vi "Unblacklist Channel.vi"(8 "error in (no error)":errorcluster, 9 "Channel 2":string, 10 "Channel 1":string, 11 "SLSC Switch in":refnum<class "SLSC Switch.lvclass">) -> (0 "error out":errorcluster, 1 "found?":bool, 3 "SLSC Switch out":refnum<class "SLSC Switch.lvclass">)   [LabVIEW 2015, in "SLSC Switch.lvclass"]
uses:
  SLSC Switch.lvclass
  SLSC Switch.lvclass/SLSC Switch.ctl
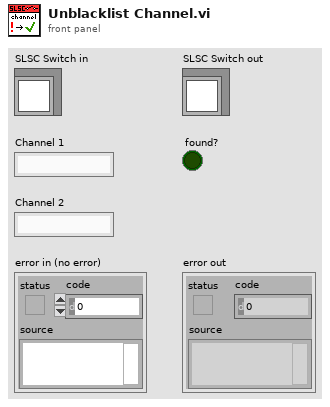
[diagram p1: front panel]
types:
  T1 = typedef "SLSC Switch.lvclass/Connection.ctl" = cluster{"channel 1":string, "channel 2":string}
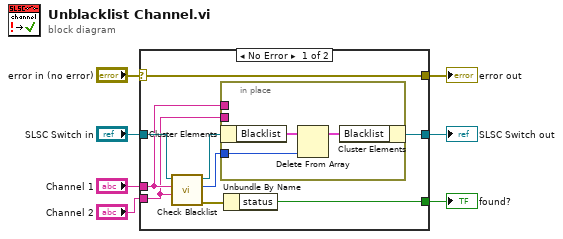
[diagram p0: block diagram]
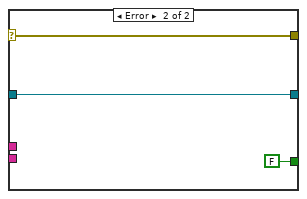
[diagram p2: hidden frame]
diagram:
  n1 = case shown="No Error" "error in (no error)" {
    selector: "error in (no error)" -> [w16 w22]
    tunnel: [w16 w22] -> w6
    tunnel: [w15 w21] -> w4
    tunnel: "SLSC Switch in" -> [w14 w21]
    tunnel: "Channel 1" -> [w12 _]
    tunnel: [w8 FALSE] -> w2
    tunnel: "Channel 2" -> [w11 _]
    frame No Error {
      n2 = call "Check Blacklist.vi"("Channel 2"=w11, "Channel 1"=w12, "SLSC Switch in"=w14) -> ("error out"=w9:errorcluster, "index"=w10:i32, "SLSC Switch out"=w13:refnum<class "SLSC Switch.lvclass">)  [unwired: 6 in]
      n3 = in-place {
        in-place-border: w12 -> [_]
        in-place-border: w11 -> [_]
        in-place-border: w10 -> [w17]
        n4 = in-place-cluster #1(w13) -> ("Blacklist"=w19:T1[])
        n5 = Delete From Array(array=w19, index=w17) -> (array with subset deleted=w18:T1[])  [unwired: 1 in, 1 out]
        n6 = in-place-cluster #1("Blacklist"=w18) -> (w15:refnum<class "SLSC Switch.lvclass">)
      }
      n7 = Unbundle By Name(w9) -> ("status"=w8:bool)
    }
    frame Error {
    }
  }
  "error out" <- w6
  "SLSC Switch out" <- w4
  "found?" <- w2
